vi "SearchForMergeIndex.vi"(10 "text":string="HEADER,TR Address, RF Direction,Select Command, Phase Shift (deg), Attenuation (dB), Temperature (C),Date,Time,\n,0,Tx,Vertical,11.250,1.000,23.3,2015/07/22,22:52:54\nFreq(Hz),S11(DB),S11(DEG),S12(DB),S12(DEG),S21(DB),S21(DEG),S22(DB),S22(DEG)\n5000000000,-42.771954,152.22778,0.082412034,-0.52403092,0.030667592,0.65514064,-48.369854,61.337074\n5005000000,-46.862316,169.26343,0.081046775,-0.41602013,0.033997945,0.62726825,-46.838844,49.065746\n5010000000,-44.007118,171.36211,0.08570607,-0.50450921,0.027771581,0.60231954,-48.501251,34.107002\n5015000000,-44.942177,170.8213,0.076357558,-0.55446047,0.02...", 11 "Step N of 131,072":i32) -> (0 "Found Match or Insert":bool, 1 "Copy":bool, 2 "incr file index":i64, 3 "copy length":i32, 4 "sweep record numbers":i32[](graph), 5 "case":u32, 6 "Timestamps":i32[](array[numeric]), 7 "ENDOFFILE":bool)   [LabVIEW 2018, in "ExistingFileMgr.lvclass"] (continued)
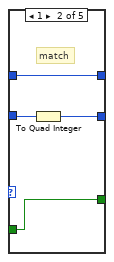
[diagram p4: hidden frame]
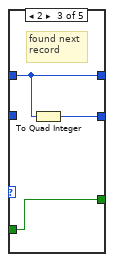
[diagram p5: hidden frame]
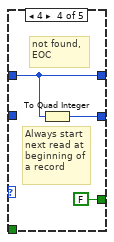
[diagram p6: hidden frame]
    n7 = Not(x=w35) -> (.not. x?=w29:bool)
    n8 = Compound Arithmetic op=OR(w30, w27, "stop") -> (w44:bool)
    "i" <- w40
  }
  "Found Match or Insert" <- w2
  "EOC" <- w11
  n9 = String Length(string="text") -> (length=→"length":i32)
  n10 = case shown="True" w11 {
    tunnel: w10 -> [w47 w57]
    tunnel: w9 -> [_ w50]
    tunnel: [w47 w55] -> w8
    tunnel: w7 -> [w46 w52]
    tunnel: [w46 w51] -> w6
    tunnel: [w45 w48] -> w4
    tunnel: w5 -> [w45 w49]
    frame False {
    }
    frame True {
      # "remove\npartial\nrecord"
      n11 = Array Subset(array=w57, index=0, length=w50) -> (w55:i32[])
      n12 = Array Subset(array=w52, index=0, length=w50) -> (w51:T2[])
      n13 = Array Subset(array=w49, index=0, length=w50) -> (w48:i32[])
    }
  }
  "Existing Sequence" <- w6
  "sweep record numbers" <- w8
  "Timestamps" <- w4
  n14 = Compound Arithmetic op=AND(w3, invert w2) -> (w1:bool)
  "ENDOFFILE" <- w1
  n15 = Build Array(w22, w21, w11, w1) -> (w20:bool[])
  n16 = Not Equal To 0?(x=w9) -> (x != 0?=w16:bool)
  n17 = Boolean Array To Number(Boolean array=w20) -> (number=w19:u32)
  "case" <- w19
  n18 = case shown="8" w19 {
    tunnel: [_ w61 w64 w67 w68] -> w18
    tunnel: [_ w60 w63 FALSE _] -> w17
    tunnel: w16 -> [_ w60 w63 _ _]
    tunnel: w15 -> [_ w58 w62 w66 _]
    tunnel: w14 -> [_ w59 _ _ w69]
    tunnel: [_ w58 w62 w66 w69] -> w13
    frame 0, Default {
    }
    frame 1 {
      # "match"
      n19 = To Quad Integer(1:w59) -> (0:w61:i64)
    }
    frame 2 {
      # "found next\nrecord"
      n20 = To Quad Integer(1:w62) -> (0:w64:i64)
    }
    frame 4 {
      # "Always start next read at beginning of a record"
      # "not found,\nEOC"
      n21 = To Quad Integer(1:w66) -> (0:w67:i64)
    }
    frame 8 {
      # "ENDOFFILE,\nno match"
      n22 = To Quad Integer(1:w69) -> (0:w68:i64)
    }
  }
  "incr file index" <- w18
  "Copy" <- w17
  "copy length" <- w13
